vi "Wait If Error(ms).vi"(7 "milliseconds to wait(100ms)":u32=100, 11 "error in (no error)":errorcluster caption="Error in (no error)") -> (8 "millisecond timer value":u32, 15 "error out":errorcluster)   [LabVIEW 2017]
doc: "Waits the given number of milliseconds and passes the error cluster through unchanged."
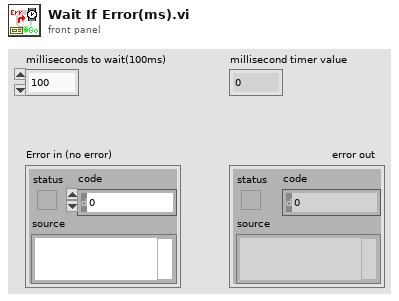
[diagram p1: front panel]
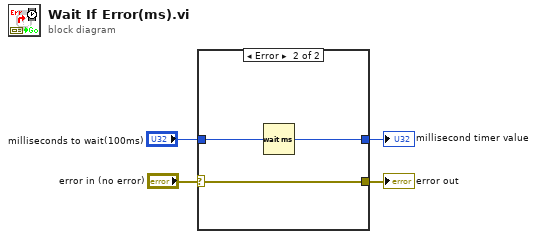
[diagram p0: block diagram]
diagram:
  n1 = case shown="Error" "error in (no error)" {
    selector: "error in (no error)" -> [w5 w6]
    tunnel: "milliseconds to wait(100ms)" -> [_ w8]
    tunnel: [_ w7] -> w3
    tunnel: [w5 w6] -> w1
    frame No Error {
    }
    frame Error {
      n2 = Wait (ms)(milliseconds to wait=w8) -> (millisecond timer value=w7:u32)
    }
  }
  "millisecond timer value" <- w3
  "error out" <- w1
